vi "QNET_ROTPEN_Digital_Scopes.vi"(1 "ROTPEN Angles":T1, 2 "Motor Speed (rad/s)":dbl, 3 "Im (A)":dbl) -> (0 "ROTPEN Digital Scopes":T2)   [LabVIEW 2021]
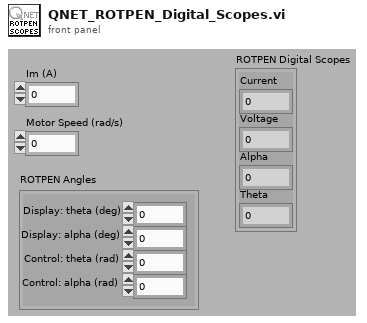
[diagram p1: front panel]
types:
  T1 = cluster{"Display: theta (deg)":dbl, "Display: alpha (deg)":dbl, "Control: alpha (rad)":dbl, "Control: theta (rad)":dbl}
  T2 = cluster{"Current":dbl, "Voltage":dbl, "Alpha":dbl, "Theta":dbl}
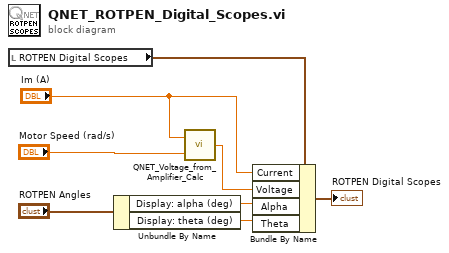
[diagram p0: block diagram]
diagram:
  n1 = local read "ROTPEN Digital Scopes"() -> (w7:T2)
  n2 = Unbundle By Name("ROTPEN Angles") -> ("Display: alpha (deg)"=w2:dbl, "Display: theta (deg)"=w1:dbl)
  n3 = call "QNET_Voltage_from_Amplifier_Calc.vi"("Speed (rad/s)"="Motor Speed (rad/s)", "Im (A)"="Im (A)") -> ("Vm (V)"=w4:dbl)
  n4 = Bundle By Name(cluster=w7, "Current"="Im (A)", "Voltage"=w4, "Alpha"=w2, "Theta"=w1) -> (→"ROTPEN Digital Scopes":T2)
